vi "Bind Integer.vi"(8 "error in (no error)":errorcluster, 10 "Integer (I64)":i64, 11 "SQL Statement in":refnum<class "SQL Statement.lvclass">) -> (0 "error out":errorcluster, 3 "SQL Statement out":refnum<class "SQL Statement.lvclass">)   [LabVIEW 2023, in "SQLite.lvlib" / "SQL Statement.lvclass"]
doc: "Binds the next parameter as an SQLite3 INTEGER datatype (equivalent to I64)."
uses:
  SQL Statement.lvclass
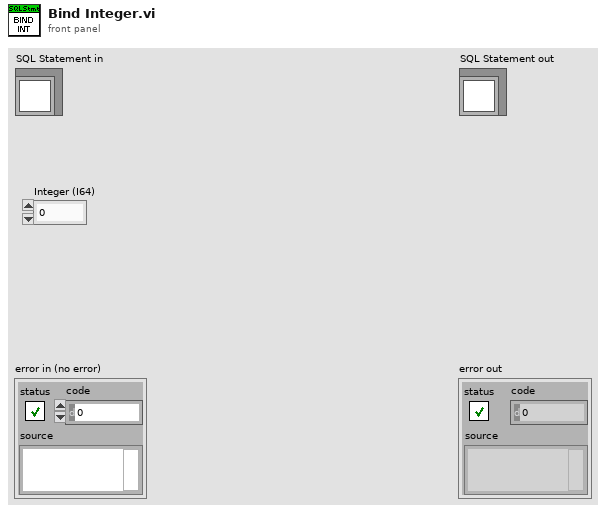
[diagram p1: front panel]
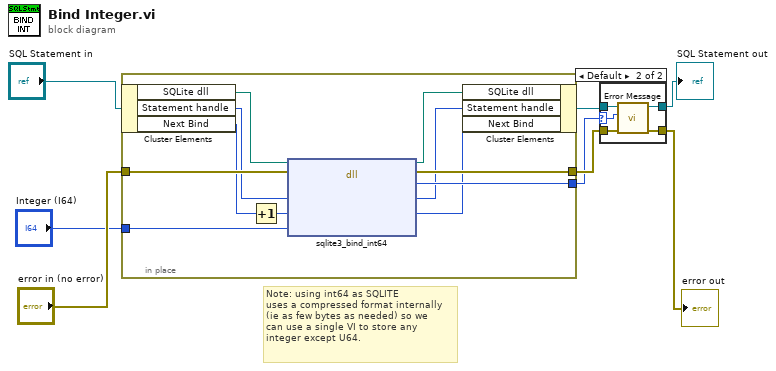
[diagram p0: block diagram]
diagram:
  # "Note: using int64 as SQLITE\nuses a compressed format internally\n(ie as few bytes as needed) so we \ncan use a single VI to store any\ninteger except U64."
  n1 = in-place {
    in-place-border: "error in (no error)" -> [w19]
    in-place-border: "Integer (I64)" -> [w18]
    in-place-border: [w17] -> w6
    in-place-border: [w16] -> w5
    n2 = in-place-cluster #1("SQL Statement in") -> ("SQLite dll"=w15:path, "Statement handle"=w12:u64, "Next Bind"=w11:i32)
    n3 = Increment(x=w11) -> (x+1=w10:i32)
    n4 = dll-call lib="C:/LabVIEW_JDP/Support/SQLite/sqlite3.dll" fn="sqlite3_bind_int64"(path in=w15, error in=w19, "Statement"=w12, "Parameter"=w10, "Integer"=w18) -> (path out=w14:path, error out=w17:errorcluster, "Result Code"=w16:i32, "Statement"=w13:u64, "Parameter"=w9:i32)  [unwired: 2 in]
    n5 = in-place-cluster #1("SQLite dll"=w14, "Statement handle"=w13, "Next Bind"=w9) -> (w2:refnum<class "SQL Statement.lvclass">)
  }
  n6 = case shown="Default" w5 {
    selector: w5 -> [_ w22]
    tunnel: w2 -> [w21 w26]
    tunnel: [w21 w25] -> w4
    tunnel: w6 -> [w20 w24]
    tunnel: [w20 w23] -> w3
    frame 0 {
      # "No Error"
    }
    frame Default {
      n7 = call "Error Message.vi"("error in (no error)"=w24, "error code"=w22, "SQL Statement In"=w26) -> ("error out"=w23:errorcluster, "SQL Statement Out"=w25:refnum<class "SQL Statement.lvclass">)  [unwired: 7 in]
    }
  }
  "error out" <- w3
  "SQL Statement out" <- w4
